vi "MQTT 5.0 Constant.vi"() -> (3 "MQTT 5.0 Constant":refnum<class "MQTTVersion50.lvclass">)   [LabVIEW 2013, in "MQTT_Control_Packets_50.lvlib" / "MQTTVersion50.lvclass"]
uses:
  MQTTVersion50.lvclass
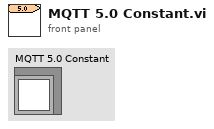
[diagram p1: front panel]
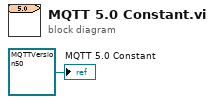
[diagram p0: block diagram]
diagram:
  "MQTT 5.0 Constant" <- refnum<class "MQTTVersion50.lvclass"> refnum ("MQTT_Control_Packets_50.lvlib:MQTTVersion50.lvclass")
